vi "NF87XX.PC get Position.vi"(0 "i ref in":refnum<vi>, 5 "error in (no error)":errorcluster) -> (14 "i ref out":refnum<vi>, 19 "error out":errorcluster)   [LabVIEW 2014, in "NF87XX.lvlib"]
doc: "This VI gets the position of the system if this is a closed loop system, and publishes the result via the DIM service <System>_Position."
uses:
  NF87XX.lvlib
  lib.lib/DimLVEvent/LVDimInterface/LVDimInterface.lvlib
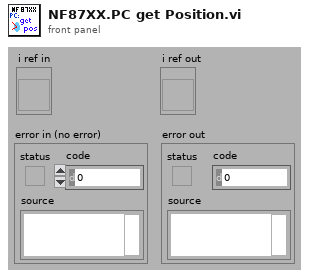
[diagram p1: front panel]
types:
  T1 = typedef "NF87XX.lvlib/NF87XX.i attribute.ctl" = cluster{"Con Settings":T2, "Drivers":T3[], "Status":cluster{"Service ID":i32, "Status":T6}, "Joystick available":bool}
  T2 = typedef "NewFocusPico.lvlib/VISA & TCPIP Control.ctl" = cluster{"VISA or TCP/IP":bool, "Init Connection":bool, "Close Connection":bool, "Resource Name":refnum<visa-resource-name>, "hostname":string, "connection ID":refnum<k5>}
  T3 = typedef "NF87XX.lvlib/NF87XX.driver Settings.ctl" = cluster{"Name":string, "Driver Type":T4, "Pico Parameter type":T5, "Acceleration [Steps/s²]":cluster{"Motor 0":dbl, "Motor 1":dbl, "Motor 2":dbl}, "Start Velocity [Steps/s]":cluster{"Motor 0":dbl, "Motor 1":dbl, "Motor 2":dbl}, "Velocity [Steps/s]":cluster{"Motor 0":dbl, "Motor 1":dbl, "Motor 2":dbl}, "axis channel":i32, "Position":i32, "Position Service ID":i32}
  T4 = typedef "NF87XX.lvlib/NF87XX.driver Type.ctl" = enum16{"not defined", "3-ch open loop drv", "1-ch closed loop drv"}
  T5 = typedef "NewFocusPico.lvlib/Pico Parameters.ctl" = cluster{"Pico Type":enum16{"Open-Loop Pico", "Close-Loop Pico", "Pico Ultra"}, "Acceleration (steps/sec^2)":string, "Velocity ( Hz)":string, "Driver":string, "Motor":string, "Channel":string, "Process Step":string}
  T6 = typedef "Status.ctl" = i16
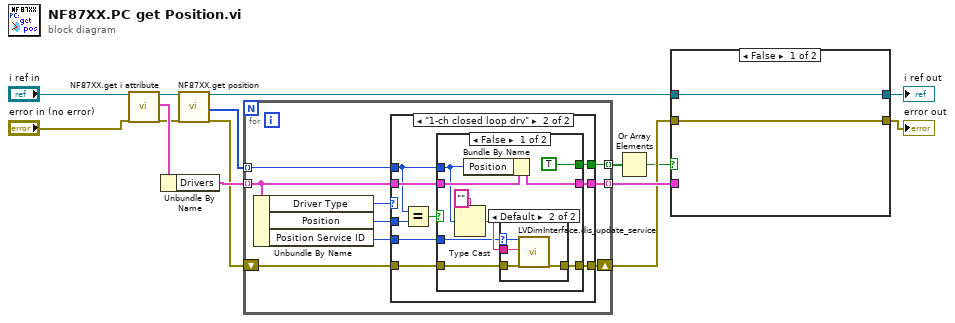
[diagram p0: block diagram]
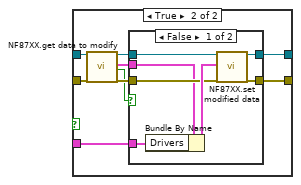
[diagram p2: hidden frame]
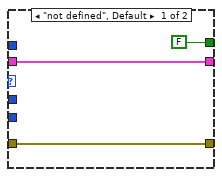
[diagram p4: hidden frame]
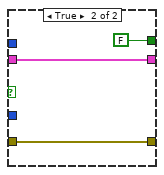
[diagram p6: hidden frame]
diagram:
  n1 = call "NF87XX.get i attribute.vi"("i ref in"="i ref in", "error in (no error)"="error in (no error)") -> ("i ref out"=w10:refnum<vi>, "i attribute"=w15:T1, "error out"=w12:errorcluster)  [unwired: 15 in]
  n2 = Unbundle By Name(w15) -> ("Drivers"=w8:T3[])
  n3 = call "NF87XX.get position.vi"("i ref in"=w10, "error in (no error)"=w12) -> ("i ref out"=w3:refnum<vi>, "Positions"=w6:i32[], "error out"=w5:errorcluster)  [unwired: 15 in]
  n4 = for {
    tunnel: w8 -> [w24] mode=indexing
    tunnel: [w23] -> w7 mode=indexing
    tunnel: w6 -> [w21] mode=indexing
    shift-right: [w19] -> w4
    shift-left: w5 -> [w20]
    tunnel: [w16] -> w2 mode=indexing
    n5 = Unbundle By Name(w24) -> ("Driver Type"=w17:T4, "Position"=w22:i32, "Position Service ID"=w18:i32)
    n6 = case shown="\"1-ch closed loop drv\"" w17 {
      tunnel: [w27 w34] -> w23
      tunnel: w24 -> [w27 w33]
      tunnel: w22 -> [_ w36]
      tunnel: w21 -> [_ w32]
      tunnel: w20 -> [w26 w31]
      tunnel: [w26 w30] -> w19
      tunnel: w18 -> [_ w29]
      tunnel: [FALSE w28] -> w16
      frame "not defined", Default {
      }
      frame "1-ch closed loop drv" {
        n7 = Equal?(x=w32, y=w36) -> (x = y?=w35:bool)
        n8 = case shown="False" w35 {
          tunnel: [w44 w53] -> w34
          tunnel: w33 -> [w45 w53]
          tunnel: w32 -> [w40 _]
          tunnel: w31 -> [w42 w52]
          tunnel: [w41 w52] -> w30
          tunnel: w29 -> [w39 _]
          tunnel: [TRUE FALSE] -> w28
          frame False {
            n9 = Type Cast(type="", x=w40) -> (*(type *) &x=w43:string)
            n10 = Bundle By Name(cluster=w45, "Position"=w40) -> (w44:T3)
            n11 = case shown="Default" w39 {
              selector: w39 -> [_ w47]
              tunnel: w43 -> [_ w50]
              tunnel: w42 -> [w46 w49]
              tunnel: [w46 w48] -> w41
              frame -1 {
              }
              frame Default {
                n12 = call "LVDimInterface.dis_update_service.vi"("my_serviceID"=w47, "data"=w50, "error in (no error)"=w49) -> ("error out"=w48:errorcluster)  [unwired: 14 in, 2 out]
              }
            }
          }
          frame True {
          }
        }
      }
    }
  }
  n13 = Or Array Elements(Boolean array=w2) -> (logical OR=w1:bool)
  n14 = case shown="False" w1 {
    tunnel: [w55 w64] -> w14
    tunnel: [w54 w63] -> w13
    tunnel: w7 -> [_ w62]
    tunnel: w4 -> [w54 w61]
    tunnel: w3 -> [w55 w59]
    frame False {
    }
    frame True {
      n15 = call "NF87XX.get data to modify.vi"("i ref in"=w59, "error in (no error)"=w61) -> ("i ref out"=w58:refnum<vi>, "i attribute"=w57:T1, "timed out"=w56:bool, "error out"=w60:errorcluster)  [unwired: 14 in]
      n16 = case shown="False" w56 {
        tunnel: [w71 w72] -> w63
        tunnel: [w70 w73] -> w64
        tunnel: w62 -> [w68 _]
        tunnel: w60 -> [w67 w72]
        tunnel: w58 -> [w66 w73]
        tunnel: w57 -> [w65 _]
        frame False {
          n17 = Bundle By Name(cluster=w65, "Drivers"=w68) -> (w69:T1)
          n18 = call "NF87XX.set modified data.vi"("i ref in"=w66, "i attribute"=w69, "error in (no error)"=w67) -> ("i ref out"=w70:refnum<vi>, "error out"=w71:errorcluster)  [unwired: 15 in]
        }
        frame True {
        }
      }
    }
  }
  "i ref out" <- w14
  "error out" <- w13
